vi "Write Index.vi"(8 "error in (no error)":errorcluster, 10 "Index":i32, 11 "CCD in":refnum<class "CCD.lvclass">) -> (0 "error out":errorcluster, 3 "CCD out":refnum<class "CCD.lvclass">)   [LabVIEW 2023, in "horiba.lvlib" / "CCD.lvclass"]
doc: "Sets the device id after init"
uses:
  CCD.lvclass
  GenericDevice/GenericDevice.lvclass
  CCD.lvclass/CCD.ctl
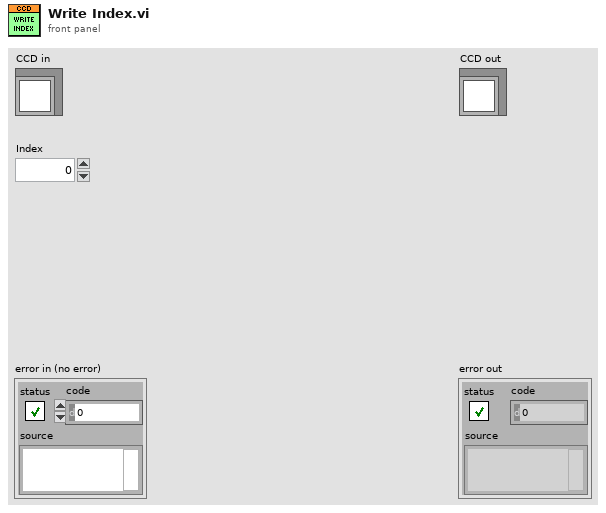
[diagram p1: front panel]
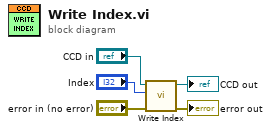
[diagram p0: block diagram]
diagram:
  n1 = call-parent "Write Index.vi"("error in (no error)"="error in (no error)", "Index"="Index", "GenericDevice in"="CCD in") -> ("error out"=→"error out":errorcluster, "GenericDevice out"=→"CCD out":refnum<class "CCD.lvclass">)  [unwired: 7 in]
